vi "MaxiGauge_Set_Status.vi"() -> ()   [LabVIEW 2020]
panel:
  out "Input":string
  in  "stop":bool
  out "Output 2":string
  in  "Delay 2":u32=500
  in  "VISA resource name":refnum<visa-resource-name>
  out "Output 1":string
  out "6":bool
  out "5":bool
  out "4":bool
  out "3":bool
  out "2":bool
  out "1":bool
  in  "Sensor 1":bool
  in  "Sensor 6":bool
  in  "Sensor 5":bool
  in  "Sensor 4":bool
  in  "Sensor 3":bool
  in  "Sensor 2":bool
  # "Should return <ACK><CR><LF>"
  # "Should return sensor 1-6 status <CR><LF>"
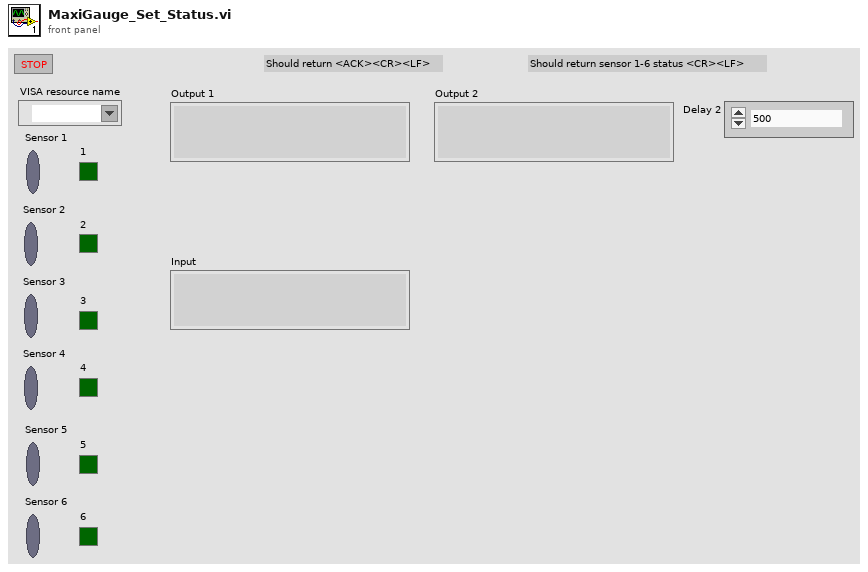
[diagram p1: front panel]
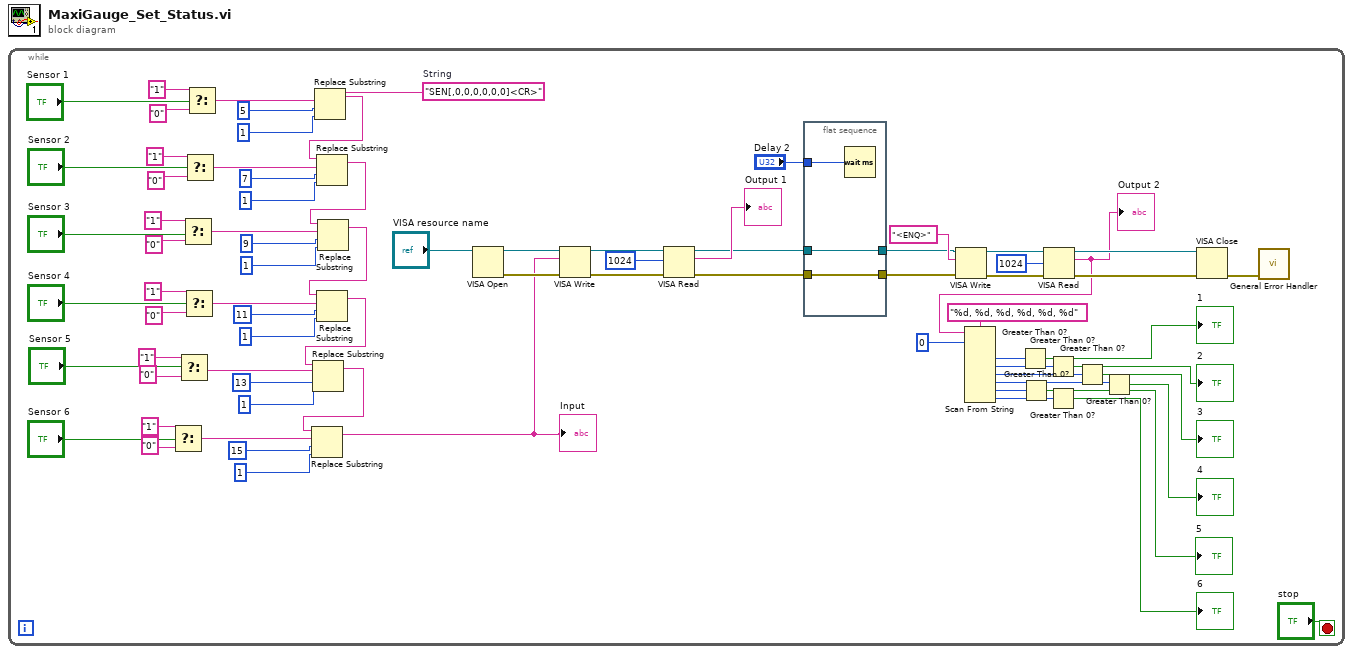
[diagram p0: block diagram]
diagram:
  n1 = while {
    stop <- "stop" stop-if-true
    w60 = "SEN[,0,0,0,0,0,0]<CR>"  # String
    n2 = Select(t="1" ("String"), s="Sensor 6", f="0" ("String")) -> (s? t:f=w38:string)
    n3 = Select(t="1" ("String"), s="Sensor 5", f="0" ("String")) -> (s? t:f=w42:string)
    n4 = Select(t="1" ("String"), s="Sensor 3", f="0" ("String")) -> (s? t:f=w50:string)
    n5 = Select(t="1" ("String"), s="Sensor 4", f="0" ("String")) -> (s? t:f=w46:string)
    n6 = Select(t="1" ("String"), s="Sensor 2", f="0" ("String")) -> (s? t:f=w54:string)
    n7 = Select(t="1" ("String"), s="Sensor 1", f="0" ("String")) -> (s? t:f=w59:string)
    n8 = Replace Substring(2:u32 1 ("unsigned 32bit integer"), 3:u32 5 ("unsigned 32bit integer"), 4:w59, 5:w60) -> (1:w53:string)  [unwired: 1 out]
    n9 = Replace Substring(2:u32 1 ("unsigned 32bit integer"), 3:u32 7 ("unsigned 32bit integer"), 4:w54, 5:w53) -> (1:w49:string)  [unwired: 1 out]
    n10 = Replace Substring(2:u32 1 ("unsigned 32bit integer"), 3:u32 9 ("unsigned 32bit integer"), 4:w50, 5:w49) -> (1:w45:string)  [unwired: 1 out]
    n11 = Replace Substring(2:u32 1 ("unsigned 32bit integer"), 3:u32 11 ("unsigned 32bit integer"), 4:w46, 5:w45) -> (1:w41:string)  [unwired: 1 out]
    n12 = Replace Substring(2:u32 1 ("unsigned 32bit integer"), 3:u32 13 ("unsigned 32bit integer"), 4:w42, 5:w41) -> (1:w37:string)  [unwired: 1 out]
    n13 = Replace Substring(2:u32 1 ("unsigned 32bit integer"), 3:u32 15 ("unsigned 32bit integer"), 4:w38, 5:w37) -> (1:w1:string)  [unwired: 1 out]
    "Input" <- w1
    n14 = VISA Open(VISA resource name="VISA resource name") -> (VISA resource name=w35:refnum<visa-resource-name>, error out=w33:errorcluster)  [unwired: 4 in]
    n15 = VISA Write(VISA resource name=w35, write buffer=w1, error in (no error)=w33) -> (VISA resource name out=w34:refnum<visa-resource-name>, error out=w32:errorcluster)  [unwired: 1 out]
    n16 = VISA Read(VISA resource name=w34, byte count=u32 1024 ("unsigned 32bit integer"), error in (no error)=w32) -> (VISA resource name out=w23:refnum<visa-resource-name>, read buffer=→"Output 1":string, error out=w22:errorcluster)  [unwired: 1 out]
    n17 = flat-sequence {
      tunnel: "Delay 2" -> [w81]
      tunnel: [w80] -> w21
      tunnel: w23 -> [w80]
      tunnel: w22 -> [w79]
      tunnel: [w79] -> w20
      frame #0 {
        n18 = Wait (ms)(milliseconds to wait=w81) -> ()  [unwired: 1 out]
      }
    }
    n19 = VISA Write(VISA resource name=w21, write buffer="<ENQ>" ("String"), error in (no error)=w20) -> (VISA resource name out=w30:refnum<visa-resource-name>, error out=w28:errorcluster)  [unwired: 1 out]
    n20 = VISA Read(VISA resource name=w30, byte count=u32 1024 ("unsigned 32bit integer"), error in (no error)=w28) -> (VISA resource name out=w19:refnum<visa-resource-name>, read buffer=w17:string, error out=w26:errorcluster)  [unwired: 1 out]
    "Output 2" <- w17
    n21 = Scan From String(format string="%d, %d, %d, %d, %d, %d", input string=w17, initial scan location=u32 0 ("unsigned 32bit integer")) -> (output 1=w14:i32, output 2=w13:i32, output 3=w12:i32, output 4=w8:i32, output 5=w6:i32, output 6=w4:i32)  [unwired: 7 in, 3 out]
    n22 = Greater Than 0?(x=w14) -> (x > 0?=→"1":bool)
    n23 = Greater Than 0?(x=w6) -> (x > 0?=→"5":bool)
    n24 = Greater Than 0?(x=w13) -> (x > 0?=→"2":bool)
    n25 = Greater Than 0?(x=w4) -> (x > 0?=→"6":bool)
    n26 = Greater Than 0?(x=w12) -> (x > 0?=→"3":bool)
    n27 = Greater Than 0?(x=w8) -> (x > 0?=→"4":bool)
    n28 = VISA Close(VISA resource name=w19, error in (no error)=w26) -> (error out=w18:errorcluster)
    n29 = call <vilib>:"General Error Handler.vi"("error in (no error)"=w18) -> ()  [unwired: 10 in, 5 out]
  }
